vi "Close Form.vi"(8 "error in (no error)":errorcluster, 10 "Form Name":T1, 11 "Form Server in":refnum<class "Form Server.lvclass">) -> (0 "error out":errorcluster, 3 "Form Server out":refnum<class "Form Server.lvclass">)   [LabVIEW 2020, in "Form Server.lvlib" / "Form Server.lvclass"]
uses:
  Form Server.lvclass
  Autoclose manager/Form ID.ctl
  Form Server.lvclass/Form Server.ctl
  Form Server Configuration/Form Server Configuration.lvclass/Form Server Configuration.ctl
  <vilib>/ActorFramework/Message Enqueuer/Message Enqueuer.lvclass/Message Enqueuer.ctl
  <vilib>/ActorFramework/Message Enqueuer/Enqueue.vi
  <vilib>/ActorFramework/Stop Msg/Stop Msg.lvclass
  C:/Program Files (x86)/National Instruments/LabVIEW 2020/vi.lib/ActorFramework/Message/Message.lvclass
  <vilib>/ActorFramework/Message Priority Queue/Priority Enqueue.vi
  Autoclose manager/Open Close Logic.lvclass
  Form Server Configuration/Form Server Configuration.lvclass
  Form Server Interfaces.lvlib
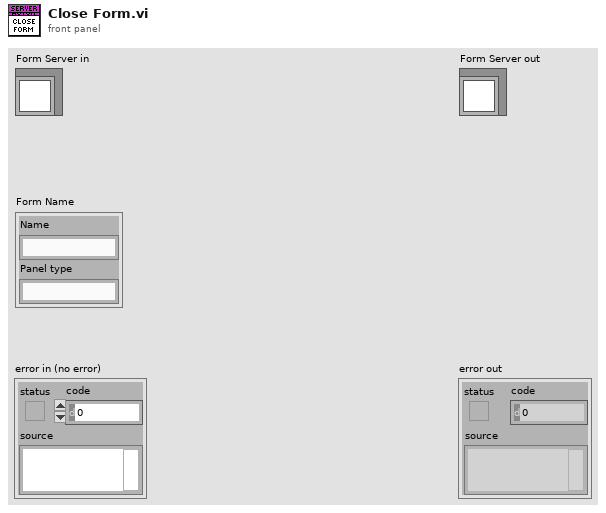
[diagram p1: front panel]
types:
  T1 = typedef "Form Server Interfaces.lvlib/Form ID.ctl" = cluster{"Name":string, "Panel type":string}
  T2 = map{T1, refnum<class "Message Enqueuer.lvclass">}
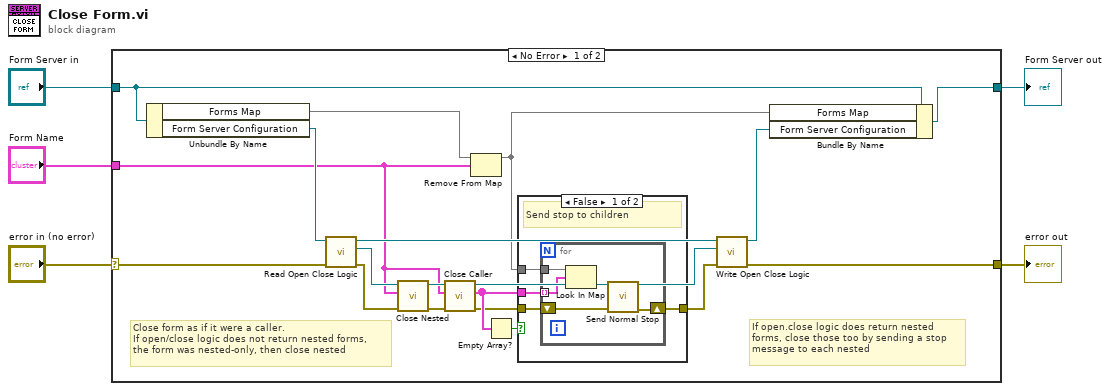
[diagram p0: block diagram]
diagram:
  n1 = case shown="No Error" "error in (no error)" {
    selector: "error in (no error)" -> [w18 w36]
    tunnel: [w14 w36] -> w4
    tunnel: [w23 w35] -> w2
    tunnel: "Form Server in" -> [w24 w35]
    tunnel: "Form Name" -> [w6 _]
    frame No Error {
      # "If open.close logic does return nested forms, close those too by sending a stop message to each nested"
      # "Close form as if it were a caller.\nIf open/close logic does not return nested forms,\nthe form was nested-only, then close nested"
      n2 = Unbundle By Name(w24) -> ("Forms Map"=w19:T2, "Form Server Configuration"=w21:refnum<class "Form Server Configuration.lvclass">)
      n3 = call "Read Open Close Logic.vi"("error in (no error)"=w18, "Form Server Configuration in"=w21) -> ("error out"=w7:errorcluster, "Form Server Interfaces.lvlib:Open Close Logic.lvclass"=w8:refnum<class "Open Close Logic.lvclass">, "Form Server Configuration out"=w16:refnum<class "Form Server Configuration.lvclass">)  [unwired: 7 in]
      n4 = call-dynamic "Close Nested.vi"("error in (no error)"=w7, "Nested"=w6, "Open Close Logic in"=w8) -> ("error out"=w9:errorcluster, "Open Close Logic out"=w10:refnum<class "Open Close Logic.lvclass">)  [unwired: 7 in]
      n5 = call-dynamic "Close Caller.vi"("error in (no error)"=w9, "Caller"=w6, "Open Close Logic in"=w10) -> ("error out"=w13:errorcluster, "Close Nested"=w20:T1[], "Open Close Logic out"=w12:refnum<class "Open Close Logic.lvclass">)  [unwired: 6 in]
      n6 = Remove From Map(10:w6, 11:w19) -> (3:w11:T2)  [unwired: 2 out]
      n7 = Empty Array?(array=w20) -> (empty?=w22:bool)
      n8 = case shown="False" w22 {
        tunnel: w20 -> [w28 _]
        tunnel: w11 -> [w27 _]
        tunnel: [w26 w34] -> w17
        tunnel: w13 -> [w25 w34]
        frame False {
          # "Send stop to children"
          n9 = for {
            tunnel: w28 -> [w32] mode=indexing
            tunnel: w27 -> [w33]
            shift-right: [w29] -> w26
            shift-left: w25 -> [w30]
            n10 = Look In Map(map=w33, key=w32) -> (value=w31:refnum<class "Message Enqueuer.lvclass">)  [unwired: 1 in, 1 out]
            n11 = call <vilib>:"Send Normal Stop.vi"("error in (no error)"=w30, "Message Enqueuer"=w31) -> ("error out"=w29:errorcluster)  [unwired: 9 in]
          }
        }
        frame True {
          # "No children forms"
        }
      }
      n12 = call "Write Open Close Logic.vi"("error in (no error)"=w17, "Form Server Interfaces.lvlib:Open Close Logic.lvclass"=w12, "Form Server Configuration in"=w16) -> ("error out"=w14:errorcluster, "Form Server Configuration out"=w15:refnum<class "Form Server Configuration.lvclass">)  [unwired: 7 in]
      n13 = Bundle By Name(cluster=w24, "Forms Map"=w11, "Form Server Configuration"=w15) -> (w23:refnum<class "Form Server.lvclass">)
    }
    frame Error {
    }
  }
  "error out" <- w4
  "Form Server out" <- w2
